vi "Gyro PID Fwd C2 Assisted Dis - Left Edge.vi"(5 "Target reflection":sgl=32.0, 6 "Target angle":sgl, 7 "Threshold to Stop":i32=1200, 8 "Threshold to slow":i32=1000, 9 "Min. speed":i32=20, 10 "Max. speed":i32=40, 11 "EV3 in":T1) -> (3 "EV3 out":T1)   [LabVIEW 2016]
uses:
  <vilib>/NXT/Subs/LVHSConnector.ctl
  <vilib>/NXT/LegoClasses/BrickReference/BrickReference.lvclass
  <vilib>/NXT/Block Support/NXT_OutputPort.ctl
  <vilib>/NXT/Block Support/NXT_InputPort.ctl
  <vilib>/NXT/NXTIO Xnodes/NXTIONodeSubVIs/LEGOResetMotors.vi
  <vilib>/NXT/Dual Mode Library/Motors/Rotation.vi
  <vilib>/NXT/NXTIO Xnodes/NXTIONodeSubVIs/NXTMotorSteeringOn.vi
  <vilib>/NXT/NXTIO Xnodes/NXTIONodeSubVIs/NXTStopMotors.vi
  <vilib>/NXT/Dual Mode Library/Waits/Wait_Num.vi
  <vilib>/NXT/NXTIO Xnodes/NXTIOXNode/NXTIO.xnode
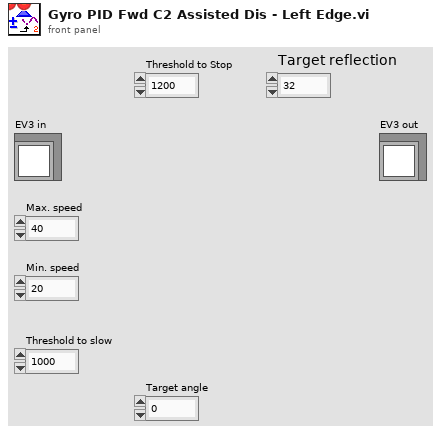
[diagram p1: front panel]
types:
  T1 = typedef "LVHSConnector.ctl" = refnum<class "BrickReference.lvclass">
  T2 = typedef "NXT_OutputPort.ctl" = u8
  T3 = typedef "NXT_InputPort.ctl" = u32
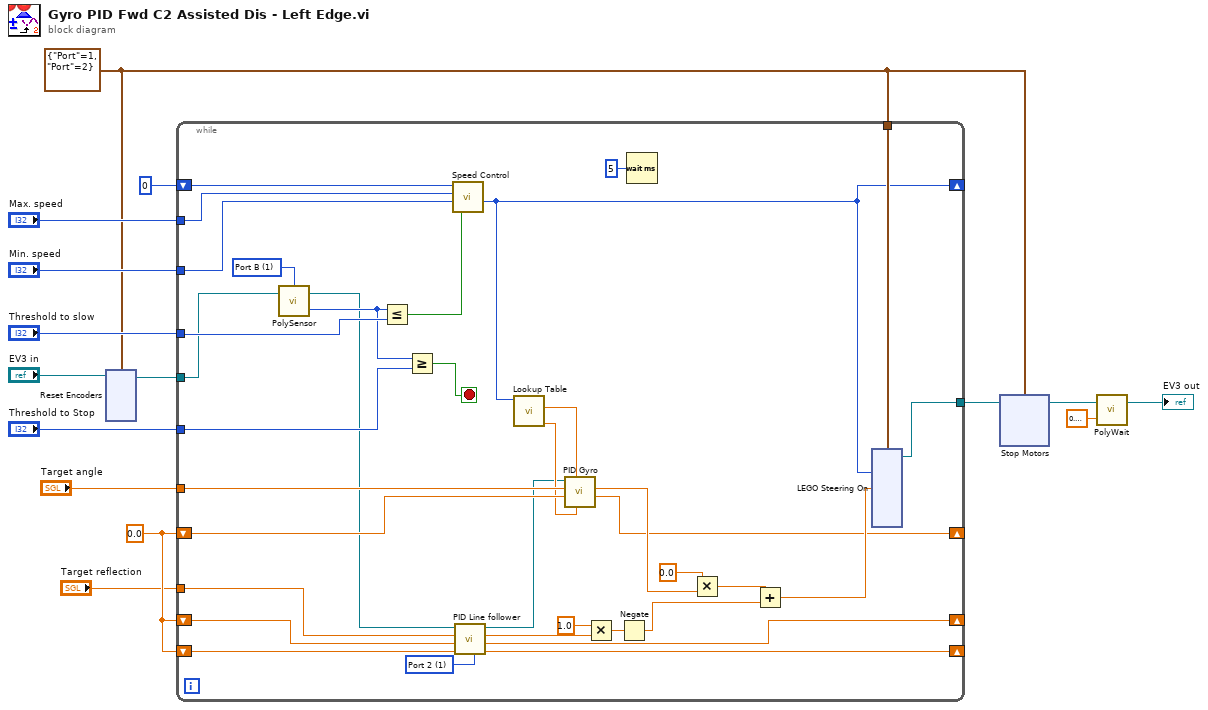
[diagram p0: block diagram]
diagram:
  w6 = cluster{"Port":T2, "Port":T2} {"Port"=1, "Port"=2} ("Motor")
  w2 = sgl 0.0
  n1 = xnode "Reset Encoders"("Motors"=w6, "NXT/EV3"="EV3 in") -> ("NXT/EV3"=w12:T1)
  n2 = while {
    tunnel: w12 -> [w41]
    shift-right: [w21] -> _
    shift-left: w2 -> [w38]
    tunnel: "Target angle" -> [w50]
    tunnel: [w47] -> w8
    tunnel: w6 -> [w49]
    shift-right: [w34] -> _
    shift-left: 0 -> [w45]
    tunnel: "Min. speed" -> [w42]
    tunnel: "Max. speed" -> [w44]
    tunnel: "Threshold to slow" -> [w43]
    tunnel: "Threshold to Stop" -> [w37]
    shift-right: [w27] -> _
    shift-left: w2 -> [w31]
    shift-right: [w28] -> _
    shift-left: w2 -> [w29]
    tunnel: "Target reflection" -> [w25]
    stop <- w16 stop-if-true
    w17 = T3 1 items=["Port 1", "Port 2", "Port 3", "Port 4"] ("Port (Port 1)")
    w48 = T2 1 items=["Port A", "Port B", "Port C", "Port D"] ("Port (Port A)")
    n3 = call-poly <vilib>:"PolySensor.vi"("NXT/EV3"=w41, "Port (Port A)"=w48) -> ("Angle of Rotation"=w39:i32, "NXT/EV3"=w24:T1)  [unwired: 1 in]
    n4 = Less Or Equal?(x=w39, y=w43) -> (x <= y?=w40:bool)
    n5 = Greater Or Equal?(x=w39, y=w37) -> (x >= y?=w16:bool)
    n6 = call "Speed Control.vi"("Speed Up or Down?"=w40, "Min. speed"=w42, "Max. speed"=w44, "Ini. speed"=w45) -> ("Speed out"=w34:i32)  [unwired: 7 in]
    n7 = call "PID Line follower.vi"("Port (Port 1)"=w17, "Old Error"=w31, "Previous integral"=w29, "Target reflection"=w25, "EV3 in"=w24) -> ("New Error"=w27:sgl, "New integral"=w28:sgl, "Total error"=w26:sgl, "EV3 out"=w30:T1)  [unwired: 3 in]
    n8 = call "Lookup Table.vi"("Speed"=w34) -> ("I"=w32:dbl, "P"=w33:dbl)  [unwired: 9 in]
    n9 = call "PID Gyro.vi"("K_i"=w32, "K_p"=w33, "Previous integral"=w38, "Target angle"=w50, "EV3 in"=w30) -> ("New integral"=w21:sgl, "Total error"=w36:sgl)  [unwired: 4 in, 1 out]
    n10 = Multiply(x=sgl 1.0, y=w26) -> (x*y=w23:sgl)
    n11 = Negate(x=w23) -> (-x=w18:sgl)
    n12 = Wait (ms)(milliseconds to wait=u32 5) -> ()  [unwired: 1 out]
    n13 = Multiply(x=sgl 0.0, y=w36) -> (x*y=w20:sgl)
    n14 = Add(x=w20, y=w18) -> (x+y=w35:sgl)
    n15 = xnode "LEGO Steering On"("Steering 1"=w35, "Power 1"=w34, "Motors"=w49) -> ("NXT/EV3"=w47:T1)  [unwired: 1 in]
  }
  n16 = xnode "Stop Motors"("Motors"=w6, "NXT/EV3"=w8) -> ("NXT/EV3"=w7:T1)
  n17 = call-poly <vilib>:"PolyWait.vi"("Time (1 sec)"=sgl 0.2, "NXT/EV3"=w7) -> ("NXT/EV3"=→"EV3 out":T1)  [unwired: 2 in]
